vi "realtime-callable-func.vi"() -> ()   [LabVIEW 2018]
uses:
  <vilib>/Platform/TimedLoop/XDataNode/timing_clust.ctl
  <vilib>/Platform/TimedLoop/XDataNode/nitl_modes.ctl
  <vilib>/Platform/TimedLoop/XDataNode/wakeup.ctl
  <vilib>/rvi/Emulation/niFpgaGetClockAttributes.vi
  <vilib>/rvi/Emulation/niFpgaSctlEmulationGetInTimedLoop.vi
  <vilib>/rvi/Emulation/niFpgaEmulationReportErrorSimple.vi
  <vilib>/rvi/Emulation/niFpgaProcessEmulError.vi
  <vilib>/rvi/Emulation/niFpgaCriticalErrorInLSC.vi
  <vilib>/Platform/TimedLoop/XDataNode/XDataNode.xnode
  <vilib>/Platform/TimedLoop/XDataNode/XDNodeRunTimeDep.lvlib
panel:
  out "x .or. y?":bool
  out "output valid":bool
  out "s? t:f":fxp<+/-,32,16>
  in  "stop":bool
  out "Output":sgl
  out "ready for input":bool
  in  "Input":fxp<+/-,32,16>
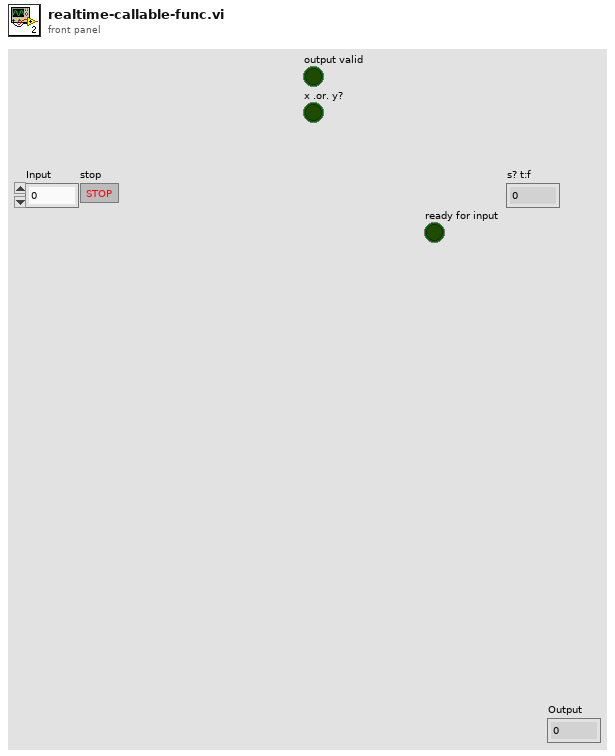
[diagram p1: front panel]
types:
  T1 = typedef "XDNodeRunTimeDep.lvlib/timing_clust.ctl" = cluster{"Expected End [f-1]":u64, "Actual End [f-1]":u64, "Finished Late? [f-1]":bool, "Expected End [i-1]":u64, "Actual End [i-1]":u64, "Finished Late? [i-1]":bool, "Expected Start [i]":u64, "Actual Start [i]":u64, "Expected Start [f]":u64, "Actual Start [f]":u64, "Source Name":string, "Structure Name":string, "Period":i64, "Deadline":i64, "Offset":i64, "Start":i64, "Priority":i32, "Timeout":i32, "Mode":T2, "Wakeup Reason":T3, "Error":errorcluster, "Source Type":string, "Secondary Source Type":string, "Global End Time":u64, "Global Start Time":u64, "Frame Duration":u64, "Iteration Duration":u64, "Assigned CPU":i32, "I/O Scan Engine Mode":u32}
  T2 = typedef "XDNodeRunTimeDep.lvlib/nitl_modes.ctl" = enum32{"No Change", "Process missed periods, maintain original phase", "Discard missed periods, maintain original phase", "Process missed periods, ignore original phase", "Discard missed periods, ignore original phase"}
  T3 = typedef "XDNodeRunTimeDep.lvlib/wakeup.ctl" = enum32{"Normal", "Aborted", "Asynchronous wakeup", "Timing source error", "Timed loop error", "Timeout"}
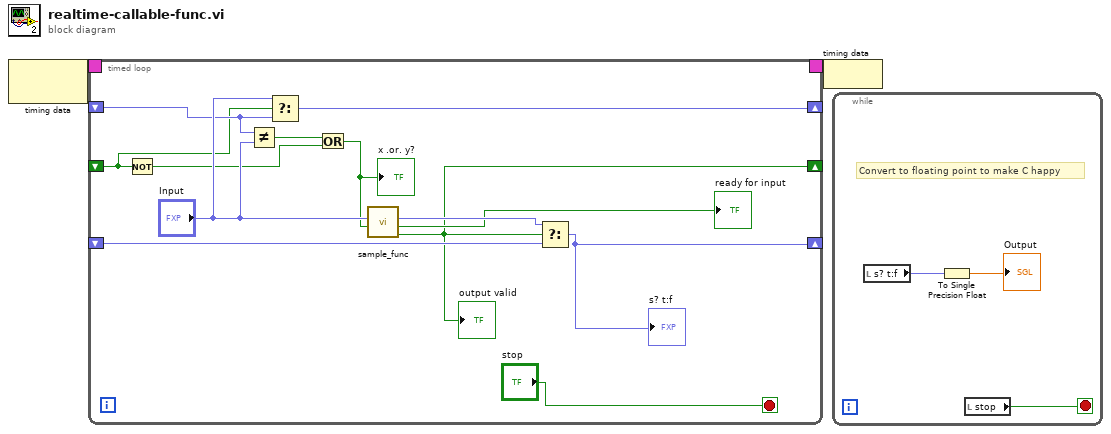
[diagram p0: block diagram]
diagram:
  n1 = node-c288() -> (w2:T1)  [unwired: 1 in]
  n2 = timed-loop {
    timing: w2 -> [_]
    timing-out: [_] -> w1
    shift-right: [w11] -> _
    shift-left: _ -> [w14]
    shift-right: [w10] -> _
    shift-left: _ -> [w8]
    shift-right: [w6] -> _
    shift-left: _ -> [w3]
    stop <- "stop" stop-if-true
    n3 = Not(x=w3) -> (.not. x?=w4:bool)
    n4 = Not Equal?(x=w8, y="Input") -> (x != y?=w7:bool)
    n5 = Select(t="Input", s=w3, f=w8) -> (s? t:f=w10:fxp<+/-,32,16>)
    n6 = Or(x=w7, y=w4) -> (x .or. y?=w5:bool)
    "x .or. y?" <- w5
    n7 = call "sample_func.vi"("ready for output (T)"=w5, "x"="Input") -> ("output valid"=w6:bool, "ready for input"=→"ready for input":bool, "Output"=w15:fxp<+/-,32,16>)  [unwired: 7 in]
    "output valid" <- w6
    n8 = Select(t=w15, s=w6, f=w14) -> (s? t:f=w11:fxp<+/-,32,16>)
    "s? t:f" <- w11
  }
  n9 = node-c288(w1) -> ()
  n10 = while {
    stop <- w19 stop-if-true
    # "Convert to floating point to make C happy"
    n11 = local read "s? t:f"() -> (w18:fxp<+/-,32,16>)
    n12 = To Single Precision Float(number=w18) -> (single precision float=→"Output":sgl)
    n13 = local read "stop"() -> (w19:bool)
  }
